vi "F Dwf Enum Analog In Bits.vi"(8 "error in (no error)":errorcluster, 10 "pnBits":i32, 11 "idxDevice":i32) -> (0 "error out":errorcluster, 2 "pnBits out":i32, 3 "function return":i32)   [LabVIEW 2019, in "Olasdwf.lvlib"]
doc: "DWFAPI int FDwfEnumAnalogInBits(int idxDevice, int *pnBits);"
uses:
  Olasdwf.lvlib
  Windows/System32/dwf.dll
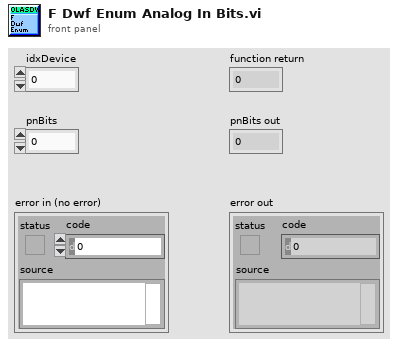
[diagram p1: front panel]
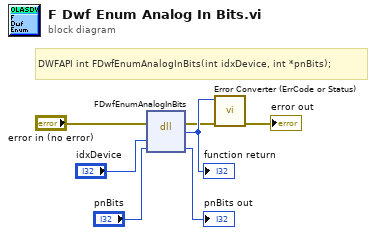
[diagram p0: block diagram]
diagram:
  # "DWFAPI int FDwfEnumAnalogInBits(int idxDevice, int *pnBits);"
  n1 = dll-call lib="C:/Windows/System32/dwf.*" fn="FDwfEnumAnalogInBits"(error in="error in (no error)", "idxDevice"="idxDevice", "pnBits"="pnBits") -> (error out=w2:errorcluster, w7:i32, "pnBits"=→"pnBits out":i32)  [unwired: 3 in, 1 out]
  "function return" <- w7
  n2 = call "Error Converter (ErrCode or Status).vi"("error in (no error)"=w2, "error code"=w7) -> ("error out"=→"error out":errorcluster)  [unwired: 9 in]
